vi "AMZ_S3_AUTH_Handle Hosting Style.vi"(9 "Bucket in":string, 11 "Path and query string in":string) -> (1 "Bucket out":string, 3 "Path and query string out":string)   [LabVIEW 2015, in "LV Interface for Amazon S3.lvlib"]
uses:
  LV Interface for Amazon S3.lvlib
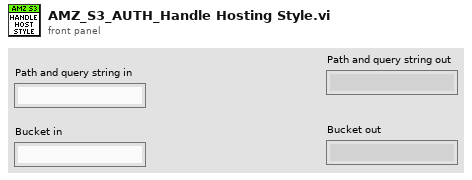
[diagram p1: front panel]
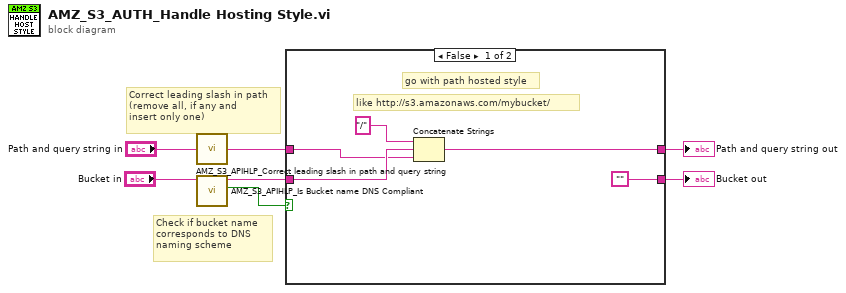
[diagram p0: block diagram]
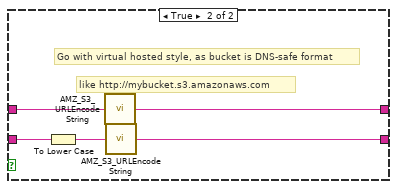
[diagram p2: hidden frame]
diagram:
  # "Correct leading slash in path\n(remove all, if any and\ninsert only one)"
  # "Check if bucket name\ncorresponds to DNS\nnaming scheme"
  n1 = call "AMZ_S3_APIHLP_Correct leading slash in path and query string.vi"("Path and query string in"="Path and query string in") -> ("Corrected Path and query string"=w4:string)  [unwired: 4 in]
  n2 = call "AMZ_S3_APIHLP_Is Bucket name DNS Compliant.vi"("Bucket in"="Bucket in") -> ("DNS Compliant?"=w1:bool, "Bucket out"=w2:string)  [unwired: 9 in]
  n3 = case shown="False" w1 {
    tunnel: w2 -> [w10 w14]
    tunnel: w4 -> [w9 w16]
    tunnel: [w12 w17] -> w7
    tunnel: ["" w15] -> w6
    frame False {
      # "like http://s3.amazonaws.com/mybucket/"
      # "go with path hosted style"
      n4 = Concatenate Strings("/" ("string"), w10, w9) -> (w12:string)
    }
    frame True {
      # "like http://mybucket.s3.amazonaws.com"
      # "Go with virtual hosted style, as bucket is DNS-safe format"
      n5 = To Lower Case(string=w14) -> (all lower case string=w13:string)
      n6 = call "AMZ_S3_URLEncode String.vi"("Unescaped string in"=w16) -> ("Escaped string out"=w17:string)  [unwired: 4 in]
      n7 = call "AMZ_S3_URLEncode String.vi"("Unescaped string in"=w13) -> ("Escaped string out"=w15:string)  [unwired: 4 in]
    }
  }
  "Path and query string out" <- w7
  "Bucket out" <- w6
